vi "C4LV_getVersions.vi"(0 "c4hdl in":refnum<k24>, 11 "error in (no error)":errorcluster) -> (4 "c4hdl out":refnum<k24>, 6 "C4HdlVersion out":string, 8 "diaphusVersion out":string, 10 "diaphusLocation out":string, 15 "error out":errorcluster)   [LabVIEW 2015, in "libC4HdlLV.lvlib"]
uses:
  libC4HdlLV.lvlib
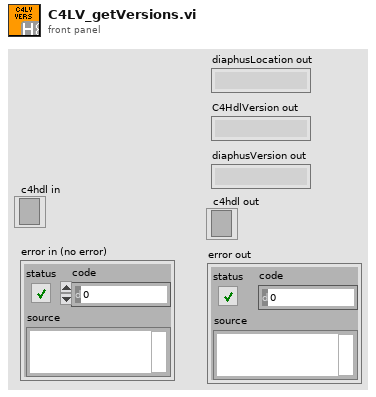
[diagram p1: front panel]
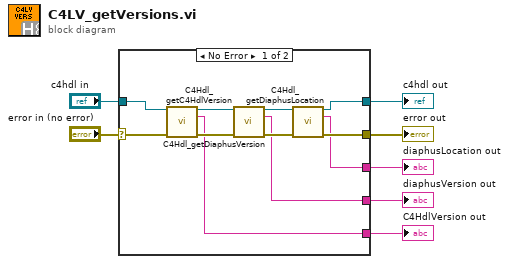
[diagram p0: block diagram]
diagram:
  n1 = case shown="No Error" "error in (no error)" {
    selector: "error in (no error)" -> [w18 w19]
    tunnel: [w15 w19] -> w6
    tunnel: "c4hdl in" -> [w14 w20]
    tunnel: [w11 w20] -> w4
    tunnel: [w10 _] -> w3
    tunnel: [w9 _] -> w2
    tunnel: [w8 _] -> w1
    frame No Error {
      n2 = call "C4Hdl_getC4HdlVersion.vi"("c4hdl in"=w14, "error in (no error)"=w18) -> ("c4hdl out"=w13:refnum<k24>, "C4HdlVersion out"=w10:string, "error out"=w17:errorcluster)  [unwired: 11 in]
      n3 = call "C4Hdl_getDiaphusVersion.vi"("c4hdl in"=w13, "error in (no error)"=w17) -> ("c4hdl out"=w12:refnum<k24>, "diaphusVersion out"=w8:string, "error out"=w16:errorcluster)  [unwired: 11 in]
      n4 = call "C4Hdl_getDiaphusLocation.vi"("c4hdl in"=w12, "error in (no error)"=w16) -> ("c4hdl out"=w11:refnum<k24>, "diaphusLocation out"=w9:string, "error out"=w15:errorcluster)  [unwired: 11 in]
    }
    frame Error {
    }
  }
  "error out" <- w6
  "c4hdl out" <- w4
  "diaphusVersion out" <- w1
  "C4HdlVersion out" <- w3
  "diaphusLocation out" <- w2
